vi "motor test.vi"(8 "error in":errorcluster) -> (0 "error out":errorcluster)   [LabVIEW 2022 SP3]
uses:
  support.project/elog/control/severity.ctl
  support.project/elog/control/category.ctl
  support.project/elog/control/type.ctl
  support.project/elog/control/logbook.ctl
  support.project/queue/Front Panel Message Queue.lvlib
  pectus/control/Param Epics Cluster.ctl
  pectus/control/cast fe motor GUI.ctl
panel:
  in  "info":bool
  out "Motor Log":string[][](array[string])
  in  "Motor On/Off":bool
  out "Info Motor":string
  in  "Motor Comands":T1
  out "Status Motor":bool
  in  "mr":bool
  in  "ma":bool
  in  "Init":bool
  in  "pos":bool
  out "Pos":dbl
  in  "Value":dbl
  in  "Device":u16(ring) items=["1"=1, "2"=2, "3"=3, "4"=4]
  in  "Card":u16(ring) items=["1"=1]
  in  "Commands":string(combo)
  in  "IOC":string(combo)
  in  "Stop":bool
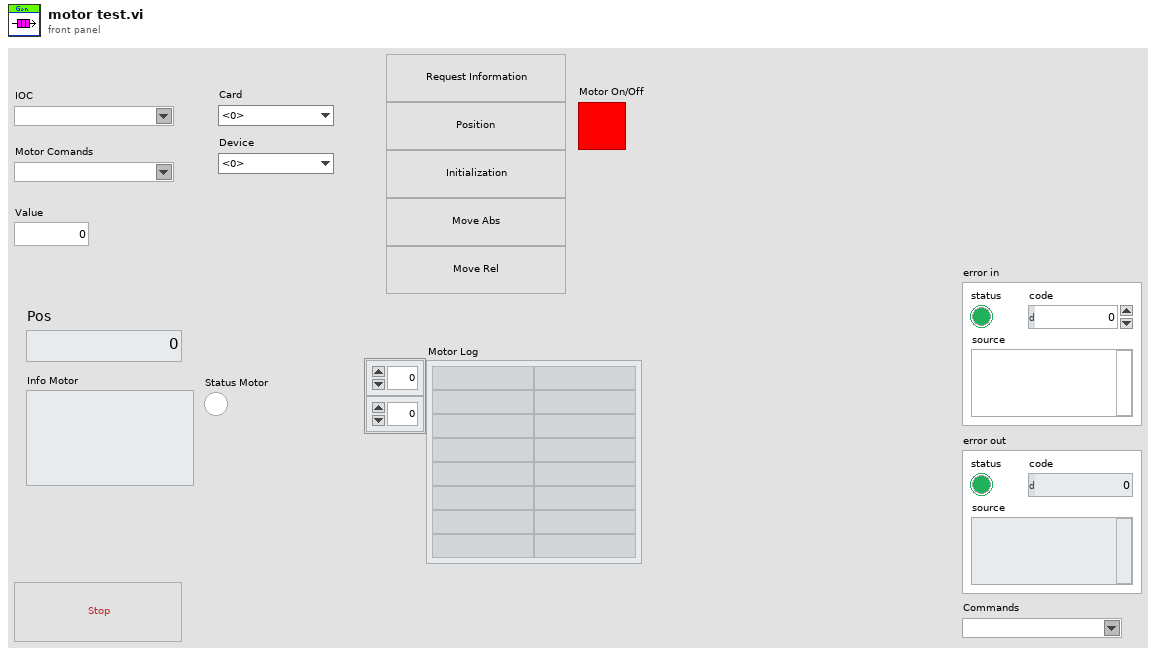
[diagram p1: front panel]
types:
  T1 = typedef "cast fe motor GUI.ctl" = string
  T2 = typedef "Front Panel Message Queue.lvlib/load Message Queues.ctl" = cluster{"Main":refnum<queue>}
  T3 = cluster{"Position Refnum":refnum<vi>, "Status Refnum":refnum<vi>, "Info Refnum":refnum<vi>}
  T4 = typedef "logbook.ctl" = string
  T5 = typedef "type.ctl" = string
  T6 = typedef "category.ctl" = string
  T7 = typedef "severity.ctl" = string
  T8 = cluster{"Logbook":T4, "Author":string, "Type":T5, "Category":T6, "Severity":T7}
  T9 = typedef "Param Epics Cluster.ctl" = cluster{"Card":u16, "Num Dev":u16}
  T10 = cluster{"IOC":string, "Command":string, "Param Cluster":T9, "value":variant}
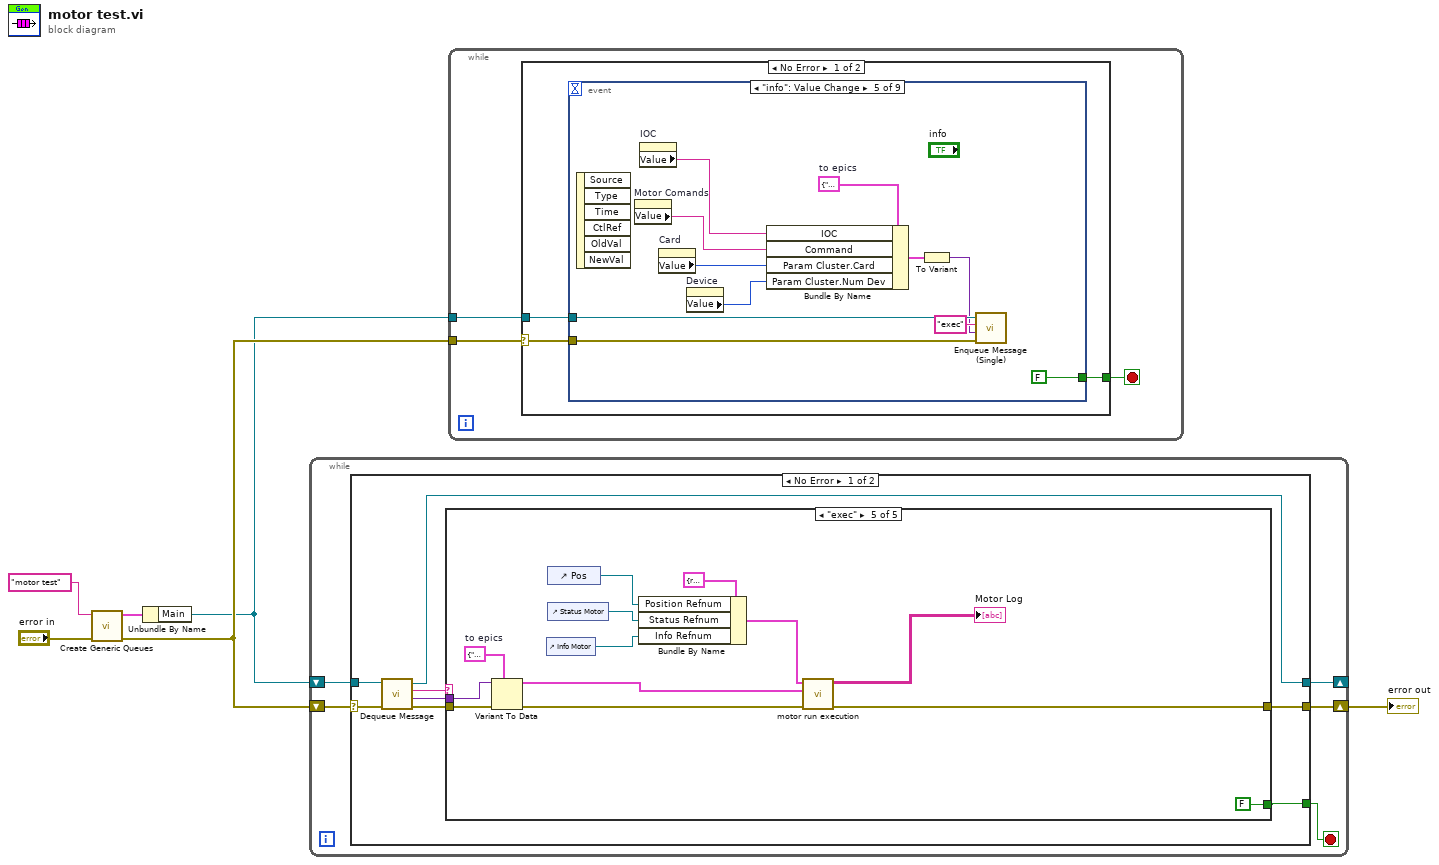
[diagram p0: block diagram]
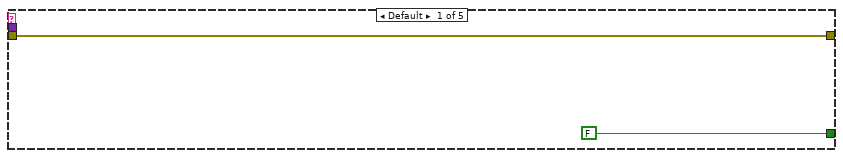
[diagram p2: hidden frame]
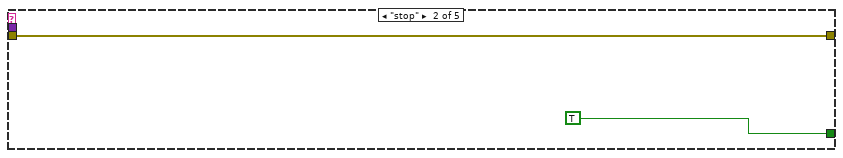
[diagram p3: hidden frame]
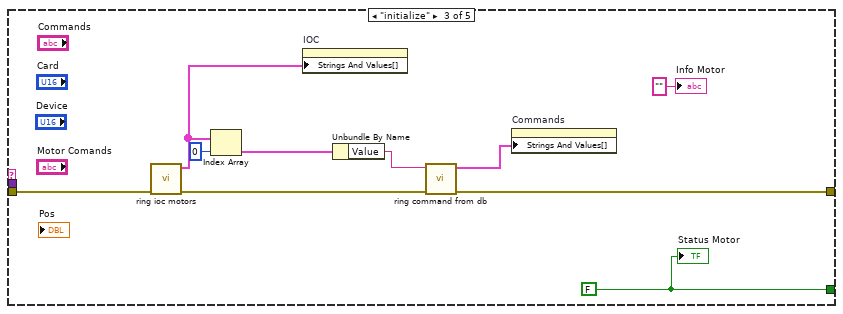
[diagram p4: hidden frame]
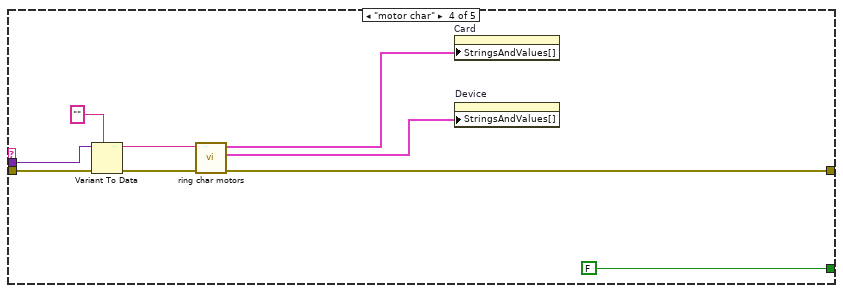
[diagram p5: hidden frame]
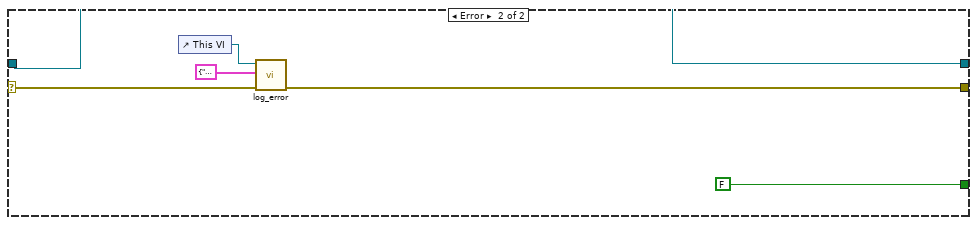
[diagram p6: hidden frame]
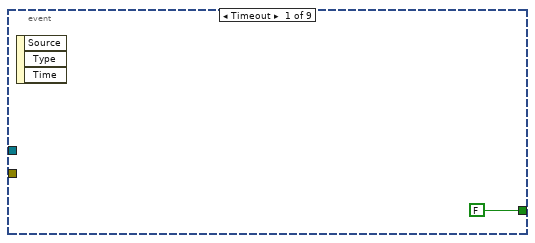
[diagram p7: hidden frame]
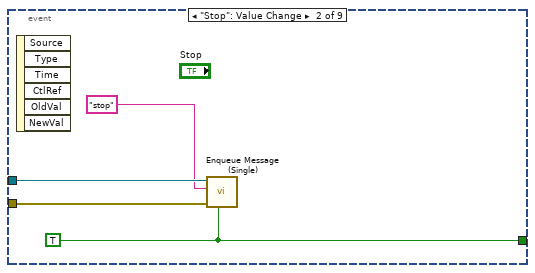
[diagram p8: hidden frame]
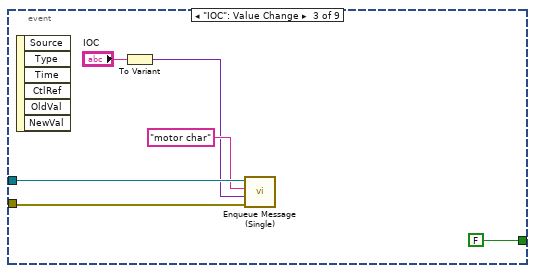
[diagram p9: hidden frame]
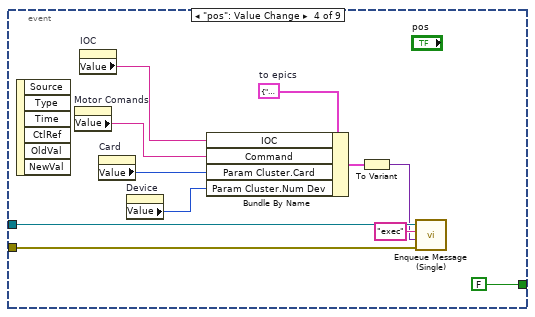
[diagram p10: hidden frame]
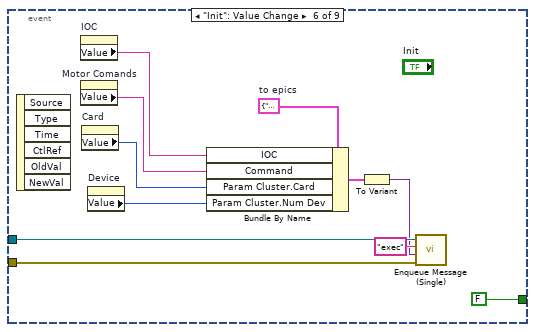
[diagram p11: hidden frame]
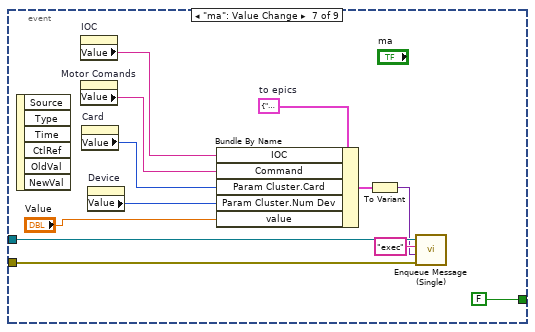
[diagram p12: hidden frame]
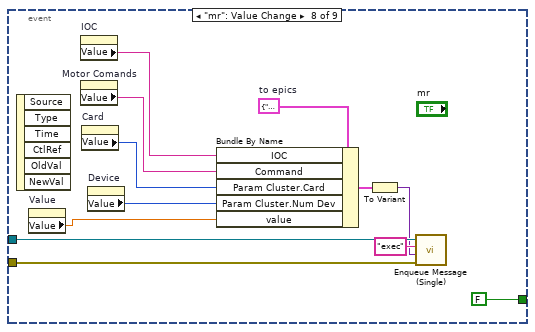
[diagram p13: hidden frame]
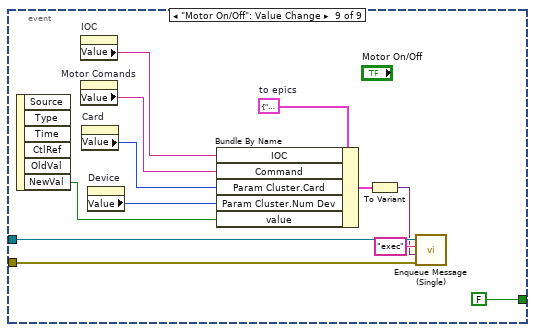
[diagram p14: hidden frame]
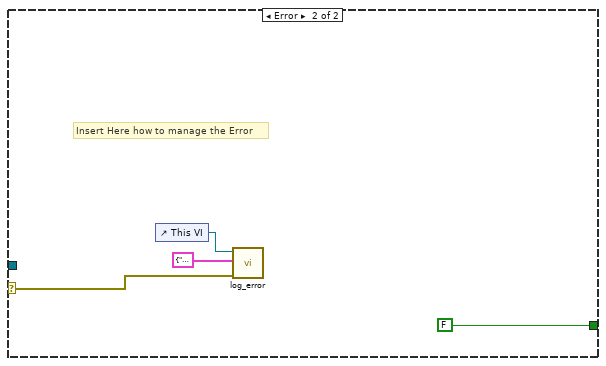
[diagram p15: hidden frame]
diagram:
  n1 = call "Create Generic Queues.vi"("error in (no error)"="error in", "name"="motor test") -> ("error out"=w3:errorcluster, "Message Queues"=w4:T2)  [unwired: 8 in]
  n2 = Unbundle By Name(w4) -> ("Main"=w2:refnum<queue>)
  n3 = while {
    shift-right: [w10] -> w1
    shift-left: w3 -> [w11]
    shift-right: [w8] -> _
    shift-left: w2 -> [w9]
    stop <- w7 stop-if-true
    n4 = case shown="No Error" w11 {
      selector: w11 -> [w19 w59]
      tunnel: [w13 w58] -> w10
      tunnel: w9 -> [w18 w57]
      tunnel: [w15 w57] -> w8
      tunnel: [w12 FALSE] -> w7
      frame No Error {
        n5 = call "Dequeue Message.vi"("error in (no error)"=w19, "Message Queue"=w18) -> ("error out"=w14:errorcluster, "Message Data"=w16:variant, "Message"=w17:string, "dup Message Queue"=w15:refnum<queue>)  [unwired: 5 in, 1 out]
        n6 = case shown="\"exec\"" w17 {
          tunnel: w16 -> [_ _ _ w39 w53]
          tunnel: w14 -> [w21 w22 w33 w40 w54]
          tunnel: [w21 w22 w31 w41 w49] -> w13
          tunnel: [FALSE TRUE w25 FALSE FALSE] -> w12
          frame Default {
          }
          frame "stop" {
          }
          frame "initialize" {
            w25 = FALSE
            n7 = call "ring ioc motors.vi"("error in"=w33) -> ("error out"=w32:errorcluster, "Strings And Values Commands"=w30:cluster{"String":string, "Value":string}[])  [unwired: 9 in]
            n8 = Index Array(array=w30, index=0) -> (element=w28:cluster{"String":string, "Value":string})
            n9 = property on="IOC" class="CmbBox"("Strings And Values[]"=w30) -> ()  [unwired: 2 in, 2 out]
            n10 = Unbundle By Name(w28) -> ("Value"=w27:string)
            n11 = call "ring command from db.vi"("error in"=w32, "IOC"=w27) -> ("error out"=w31:errorcluster, "Strings And Values Commands"=w26:cluster{"String":string, "Value":string}[])  [unwired: 8 in]
            n12 = property on="Commands" class="CmbBox"("Strings And Values[]"=w26) -> ()  [unwired: 2 in, 2 out]
            "Status Motor" <- w25
            "Info Motor" <- "" ("Info Motor")
          }
          frame "motor char" {
            n13 = Variant To Data(error in=w40, type="", Variant=w39) -> (data=w37:string, error out=w36:errorcluster)
            n14 = call "ring char motors.vi"("error in"=w36, "IOC"=w37) -> ("error out"=w41:errorcluster, "Strings And Values Device"=w34:cluster{"String":string, "Value":u16}[], "Strings And Values Card"=w35:cluster{"String":string, "Value":u16}[])  [unwired: 7 in]
            n15 = property on="Card" class="Ring (strict)"("StringsAndValues[]"=w35) -> ()  [unwired: 2 in, 2 out]
            n16 = property on="Device" class="Ring (strict)"("StringsAndValues[]"=w34) -> ()  [unwired: 2 in, 2 out]
          }
          frame "exec" {
            w50 = T10 {"IOC"="", "Command"="", "Param Cluster"={"Card"=1, "Num Dev"=1}, "value"=variant}  # to epics
            n17 = Variant To Data(error in=w54, type=w50, Variant=w53) -> (data=w51:T10, error out=w52:errorcluster)
            n18 = control-ref of="Info Motor"() -> (w45:refnum<vi>)
            n19 = control-ref of="Pos"() -> (w47:refnum<vi>)
            n20 = control-ref of="Status Motor"() -> (w46:refnum<vi>)
            n21 = Bundle By Name(cluster=T3 {"Position Refnum"=refnum, "Status Refnum"=refnum, "Info Refnum"=refnum} ("Refnum Cluster Motor"), "Position Refnum"=w47, "Status Refnum"=w46, "Info Refnum"=w45) -> (w48:T3)
            n22 = call "motor run execution.vi"("error in"=w52, "data"=w51, "Refnum Cluster Motor"=w48) -> ("error out"=w49:errorcluster, "Motor Log"=→"Motor Log":string[][])  [unwired: 6 in, 1 out]
          }
        }
      }
      frame Error {
        n23 = control-ref of="This VI"() -> (w60:refnum<vi>)
        n24 = call "log_error.vi"("error in"=w59, "Elog Properties"=T8 {"Logbook"="Error", "Author"="User", "Type"="Experiment", "Category"="General", "Severity"="Error"}, "VI Refnum"=w60) -> ("error out"=w58:errorcluster)  [unwired: 8 in]
      }
    }
  }
  "error out" <- w1
  n25 = while {
    tunnel: w3 -> [w63]
    tunnel: w2 -> [w62]
    stop <- w64 stop-if-true
    n26 = case shown="No Error" w63 {
      selector: w63 -> [w65 w150]
      tunnel: [w67 FALSE ("Stop")] -> w64
      tunnel: w62 -> [w66 _]
      frame No Error {
        n27 = event shown="[4] \"info\": Value Change" {
          selector: _ -> [_ _ _ _ _ _ _ _ _]
          dyn-events: _ -> [_ _ _ _ _ _ _ _ _]
          timeout: _ -> [_ _ _ _ _ _ _ _ _]
          tunnel: [FALSE ("Stop") w70 FALSE ("Stop") FALSE ("Stop") FALSE ("Stop") FALSE ("Stop") FALSE ("Stop") FALSE ("Stop") FALSE ("Stop")] -> w67
          tunnel: w66 -> [_ w72 w76 w87 w98 w109 w121 w133 w145]
          tunnel: w65 -> [_ w69 w77 w88 w99 w110 w122 w134 w146]
          event Timeout {
            n28 = event-data() -> ()  [unwired: 1 in, 3 out]
          }
          event "Stop": Value Change {
            w70 = TRUE ("Stop")
            n29 = event-data() -> ()  [unwired: 1 in, 6 out]
            n30 = call "Enqueue Message (Single).vi"("Priority Message? (F)"=w70, "error in (no error)"=w69, "Message"="stop", "Message Queue"=w72) -> ()  [unwired: 6 in, 2 out]
          }
          event "IOC": Value Change {
            n31 = event-data() -> ()  [unwired: 1 in, 6 out]
            n32 = To Variant(anything="IOC") -> (Variant=w73:variant)
            n33 = call "Enqueue Message (Single).vi"("error in (no error)"=w77, "Message Data"=w73, "Message"="motor char", "Message Queue"=w76) -> ()  [unwired: 6 in, 2 out]
          }
          event "pos": Value Change {
            w85 = T10 {"IOC"="", "Command"="", "Param Cluster"={"Card"=1, "Num Dev"=1}, "value"=variant}  # to epics
            n34 = event-data() -> ()  [unwired: 1 in, 6 out]
            n35 = property on="Motor Comands" class="CmbBox (strict)"() -> ("Value"=w79:T1)  [unwired: 2 in, 2 out]
            n36 = property on="IOC" class="CmbBox"() -> ("Value"=w82:string)  [unwired: 2 in, 2 out]
            n37 = property on="Card" class="Ring (strict)"() -> ("Value"=w83:u16)  [unwired: 2 in, 2 out]
            n38 = property on="Device" class="Ring (strict)"() -> ("Value"=w84:u16)  [unwired: 2 in, 2 out]
            n39 = Bundle By Name(cluster=w85, "IOC"=w82, "Command"=w79, "Param Cluster.Card"=w83, "Param Cluster.Num Dev"=w84) -> (w81:T10)
            n40 = To Variant(anything=w81) -> (Variant=w80:variant)
            n41 = call "Enqueue Message (Single).vi"("error in (no error)"=w88, "Message Data"=w80, "Message"="exec", "Message Queue"=w87) -> ()  [unwired: 6 in, 2 out]
          }
          event "info": Value Change {
            w96 = T10 {"IOC"="", "Command"="", "Param Cluster"={"Card"=1, "Num Dev"=1}, "value"=variant}  # to epics
            n42 = event-data() -> ()  [unwired: 1 in, 6 out]
            n43 = property on="Motor Comands" class="CmbBox (strict)"() -> ("Value"=w90:T1)  [unwired: 2 in, 2 out]
            n44 = property on="IOC" class="CmbBox"() -> ("Value"=w93:string)  [unwired: 2 in, 2 out]
            n45 = property on="Card" class="Ring (strict)"() -> ("Value"=w94:u16)  [unwired: 2 in, 2 out]
            n46 = property on="Device" class="Ring (strict)"() -> ("Value"=w95:u16)  [unwired: 2 in, 2 out]
            n47 = Bundle By Name(cluster=w96, "IOC"=w93, "Command"=w90, "Param Cluster.Card"=w94, "Param Cluster.Num Dev"=w95) -> (w92:T10)
            n48 = To Variant(anything=w92) -> (Variant=w91:variant)
            n49 = call "Enqueue Message (Single).vi"("error in (no error)"=w99, "Message Data"=w91, "Message"="exec", "Message Queue"=w98) -> ()  [unwired: 6 in, 2 out]
          }
          event "Init": Value Change {
            w107 = T10 {"IOC"="", "Command"="", "Param Cluster"={"Card"=1, "Num Dev"=1}, "value"=variant}  # to epics
            n50 = event-data() -> ()  [unwired: 1 in, 6 out]
            n51 = property on="IOC" class="CmbBox"() -> ("Value"=w104:string)  [unwired: 2 in, 2 out]
            n52 = property on="Motor Comands" class="CmbBox (strict)"() -> ("Value"=w101:T1)  [unwired: 2 in, 2 out]
            n53 = property on="Card" class="Ring (strict)"() -> ("Value"=w105:u16)  [unwired: 2 in, 2 out]
            n54 = property on="Device" class="Ring (strict)"() -> ("Value"=w106:u16)  [unwired: 2 in, 2 out]
            n55 = Bundle By Name(cluster=w107, "IOC"=w104, "Command"=w101, "Param Cluster.Card"=w105, "Param Cluster.Num Dev"=w106) -> (w103:T10)
            n56 = To Variant(anything=w103) -> (Variant=w102:variant)
            n57 = call "Enqueue Message (Single).vi"("error in (no error)"=w110, "Message Data"=w102, "Message"="exec", "Message Queue"=w109) -> ()  [unwired: 6 in, 2 out]
          }
          event "ma": Value Change {
            w119 = T10 {"IOC"="", "Command"="", "Param Cluster"={"Card"=1, "Num Dev"=1}, "value"=variant}  # to epics
            n58 = event-data() -> ()  [unwired: 1 in, 6 out]
            n59 = property on="IOC" class="CmbBox"() -> ("Value"=w116:string)  [unwired: 2 in, 2 out]
            n60 = property on="Motor Comands" class="CmbBox (strict)"() -> ("Value"=w113:T1)  [unwired: 2 in, 2 out]
            n61 = property on="Card" class="Ring (strict)"() -> ("Value"=w117:u16)  [unwired: 2 in, 2 out]
            n62 = property on="Device" class="Ring (strict)"() -> ("Value"=w118:u16)  [unwired: 2 in, 2 out]
            n63 = Bundle By Name(cluster=w119, "IOC"=w116, "Command"=w113, "Param Cluster.Card"=w117, "Param Cluster.Num Dev"=w118, "value"="Value") -> (w115:T10)
            n64 = To Variant(anything=w115) -> (Variant=w114:variant)
            n65 = call "Enqueue Message (Single).vi"("error in (no error)"=w122, "Message Data"=w114, "Message"="exec", "Message Queue"=w121) -> ()  [unwired: 6 in, 2 out]
          }
          event "mr": Value Change {
            w131 = T10 {"IOC"="", "Command"="", "Param Cluster"={"Card"=1, "Num Dev"=1}, "value"=variant}  # to epics
            n66 = event-data() -> ()  [unwired: 1 in, 6 out]
            n67 = property on="Value" class="DigNum (strict)"() -> ("Value"=w124:dbl)  [unwired: 2 in, 2 out]
            n68 = property on="IOC" class="CmbBox"() -> ("Value"=w128:string)  [unwired: 2 in, 2 out]
            n69 = property on="Motor Comands" class="CmbBox (strict)"() -> ("Value"=w125:T1)  [unwired: 2 in, 2 out]
            n70 = property on="Card" class="Ring (strict)"() -> ("Value"=w129:u16)  [unwired: 2 in, 2 out]
            n71 = property on="Device" class="Ring (strict)"() -> ("Value"=w130:u16)  [unwired: 2 in, 2 out]
            n72 = Bundle By Name(cluster=w131, "IOC"=w128, "Command"=w125, "Param Cluster.Card"=w129, "Param Cluster.Num Dev"=w130, "value"=w124) -> (w127:T10)
            n73 = To Variant(anything=w127) -> (Variant=w126:variant)
            n74 = call "Enqueue Message (Single).vi"("error in (no error)"=w134, "Message Data"=w126, "Message"="exec", "Message Queue"=w133) -> ()  [unwired: 6 in, 2 out]
          }
          event "Motor On/Off": Value Change {
            w143 = T10 {"IOC"="", "Command"="", "Param Cluster"={"Card"=1, "Num Dev"=1}, "value"=variant}  # to epics
            n75 = event-data() -> ("NewVal"=w136:bool)  [unwired: 1 in, 5 out]
            n76 = property on="IOC" class="CmbBox"() -> ("Value"=w140:string)  [unwired: 2 in, 2 out]
            n77 = property on="Motor Comands" class="CmbBox (strict)"() -> ("Value"=w137:T1)  [unwired: 2 in, 2 out]
            n78 = property on="Card" class="Ring (strict)"() -> ("Value"=w141:u16)  [unwired: 2 in, 2 out]
            n79 = property on="Device" class="Ring (strict)"() -> ("Value"=w142:u16)  [unwired: 2 in, 2 out]
            n80 = Bundle By Name(cluster=w143, "IOC"=w140, "Command"=w137, "Param Cluster.Card"=w141, "Param Cluster.Num Dev"=w142, "value"=w136) -> (w139:T10)
            n81 = To Variant(anything=w139) -> (Variant=w138:variant)
            n82 = call "Enqueue Message (Single).vi"("error in (no error)"=w146, "Message Data"=w138, "Message"="exec", "Message Queue"=w145) -> ()  [unwired: 6 in, 2 out]
          }
        }
      }
      frame Error {
        # "Insert Here how to manage the Error"
        n83 = control-ref of="This VI"() -> (w149:refnum<vi>)
        n84 = call "log_error.vi"("error in"=w150, "Elog Properties"=T8 {"Logbook"="Error", "Author"="User", "Type"="Experiment", "Category"="General", "Severity"="Error"}, "VI Refnum"=w149) -> ()  [unwired: 8 in, 1 out]
      }
    }
  }
